vi "Group Time To Freq.vi"(1 "Group Time":u16) -> (0 "Frequency (Hz)":dbl)   [LabVIEW 2019]
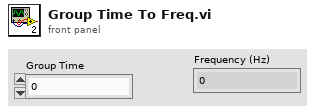
[diagram p1: front panel]
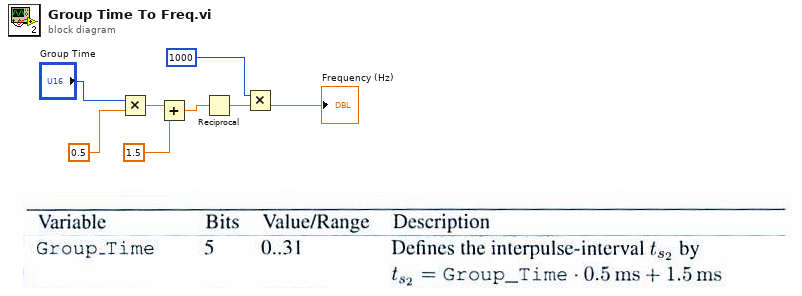
[diagram p0: block diagram]
diagram:
  n1 = Multiply(x="Group Time", y=0.5) -> (x*y=w2:dbl)
  n2 = Add(x=w2, y=1.5) -> (x+y=w5:dbl)
  n3 = Reciprocal(x=w5) -> (1/x=w6:dbl)
  n4 = Multiply(x=1000, y=w6) -> (x*y=→"Frequency (Hz)":dbl)
